vi "resamplingCore.vi"(7 "Stereo":bool, 8 "error in":errorcluster, 10 "writePath":path=path "C:/Users/tbone/Documents/GitHub/Nutella-Tsunami-Wav-Converter/convertedSamples/529 mySample.wav", 11 "readPath":path=path "C:/Users/tbone/Documents/GitHub/Nutella-Tsunami-Wav-Converter/rawSamples/CR8K/CR8KBASS.WAV") -> (0 "error out":errorcluster)   [LabVIEW 2019]
uses:
  <vilib>/sound2/lvsound2.llb/Sound Data Format.ctl
  <vilib>/sound2/lvsound2.llb/Sound File Info (path).vi
panel:
  out "sound format OUT":T1={"sample rate (S/s)"=44100.0, "number of channels"=1, "bits per sample"=16}
  out "sound format IN":T1={"sample rate (S/s)"=44100.0, "number of channels"=1, "bits per sample"=16}
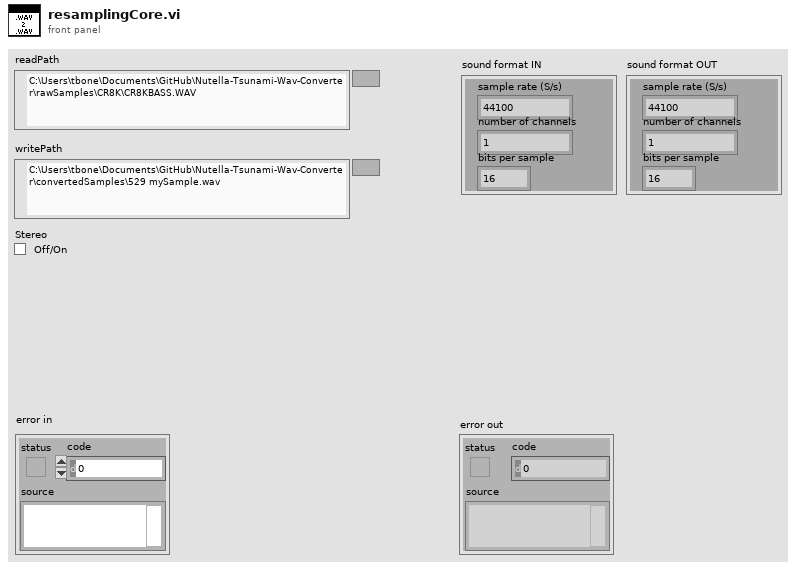
[diagram p1: front panel]
types:
  T1 = typedef "Sound Data Format.ctl" = cluster{"sample rate (S/s)":dbl, "number of channels":i32, "bits per sample":i32}
  T2 = cluster{"sound quality":enum16{"mono", "stereo"}, "rate":u32}
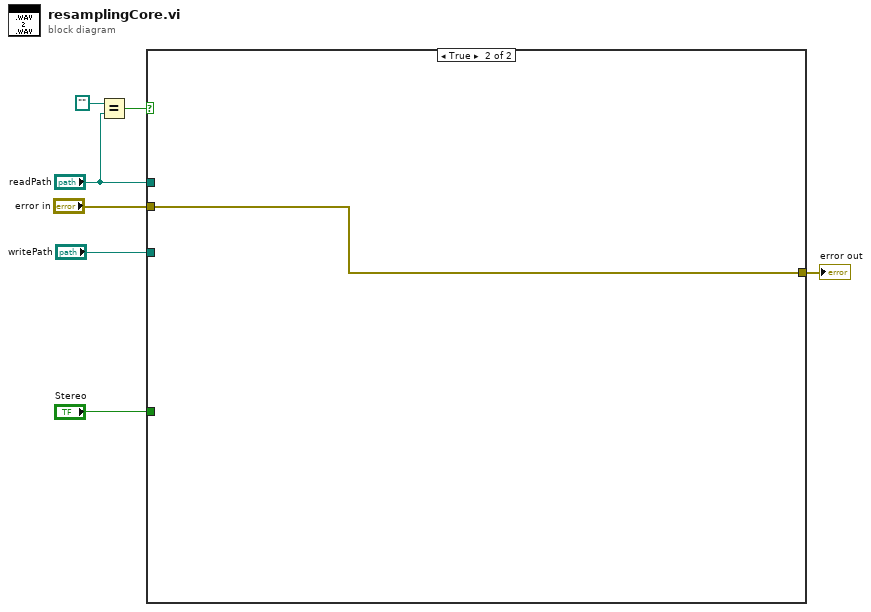
[diagram p0: block diagram]
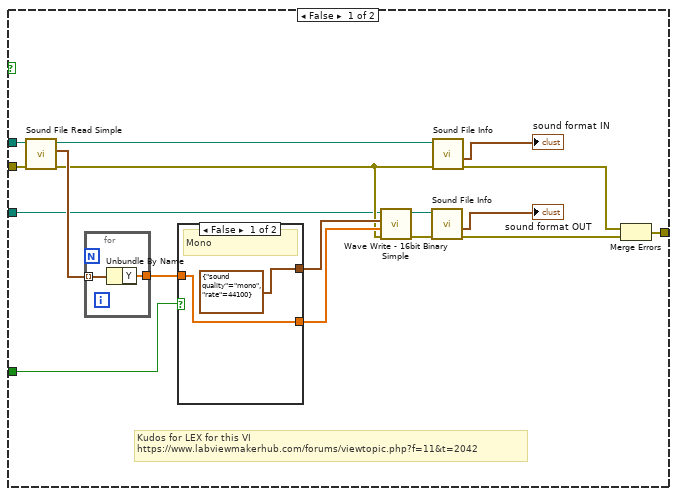
[diagram p2: hidden frame]
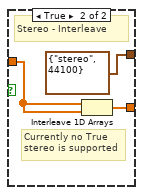
[diagram p3: hidden frame]
diagram:
  n1 = Equal?(x=path "", y="readPath") -> (x = y?=w3:bool)
  n2 = case shown="True" w3 {
    tunnel: "error in" -> [w24 w32]
    tunnel: "readPath" -> [w23 _]
    tunnel: [w20 w32] -> w6
    tunnel: "Stereo" -> [w13 _]
    tunnel: "writePath" -> [w8 _]
    frame False {
      # "Kudos for LEX for this VI\nhttps://www.labviewmakerhub.com/forums/viewtopic.php?f=11&t=2042"
      n3 = call <vilib>:"Sound File Read Simple.vi"("error in (no error)"=w24, "path"=w23) -> ("error out"=w9:errorcluster, "data"=w17:waveform(dbl)[], "path out"=w18:path)  [unwired: 6 in, 1 out]
      n4 = for {
        tunnel: w17 -> [w31] mode=indexing
        tunnel: [w30] -> w11
        n5 = Unbundle By Name(w31) -> ("Y"=w30:dbl[])
      }
      n6 = case shown="False" w13 {
        tunnel: [w26 w29] -> w12
        tunnel: w11 -> [w26 w28]
        tunnel: [T2 {"sound quality"=enum."mono", "rate"=44100} ("Sound Format") T2 {"sound quality"=enum."stereo", "rate"=44100} ("Sound Format")] -> w10
        frame False {
          # "Mono"
        }
        frame True {
          # "Currently no True \nstereo is supported"
          # "Stereo - Interleave"
          n7 = Interleave 1D Arrays(w28, w28) -> (w29:dbl[])
        }
      }
      n8 = call "Wave Write - 16bit Binary Simple.vi"("error in"=w9, "Audio Input (+/- 1)"=w12, "Sound Format"=w10, "File Path"=w8) -> ("error out"=w16:errorcluster, "File Path Out"=w14:path)  [unwired: 6 in]
      n9 = call-poly <vilib>:"Sound File Info.vi"("error in (no error)"=w16, "path"=w14) -> ("error out"=w15:errorcluster, "sound format"=→"sound format OUT":T1)  [unwired: 6 in, 2 out]
      n10 = call-poly <vilib>:"Sound File Info.vi"("error in (no error)"=w9, "path"=w18) -> ("error out"=w19:errorcluster, "sound format"=→"sound format IN":T1)  [unwired: 6 in, 2 out]
      n11 = Merge Errors(w19, w15) -> (w20:errorcluster)
    }
    frame True {
    }
  }
  "error out" <- w6
